vi "Add Output.vi"(0 "PainOutputTerminal in":refnum<class "PainOutputTerminal.lvclass">, 5 "Comiplation message":T1[](array[typedef]), 11 "error in (no error)":errorcluster) -> (4 "PainOutputTerminal out":refnum<class "PainOutputTerminal.lvclass">, 15 "error out":errorcluster)   [LabVIEW 2019, in "PainOutputTerminal.lvclass"]
uses:
  PainOutputTerminal.lvclass
  common/function utils/Validate_message.ctl
  common/function utils/Validate_MessageStatus.ctl
  PainOutputTerminal.lvclass/PainOutputTerminal.ctl
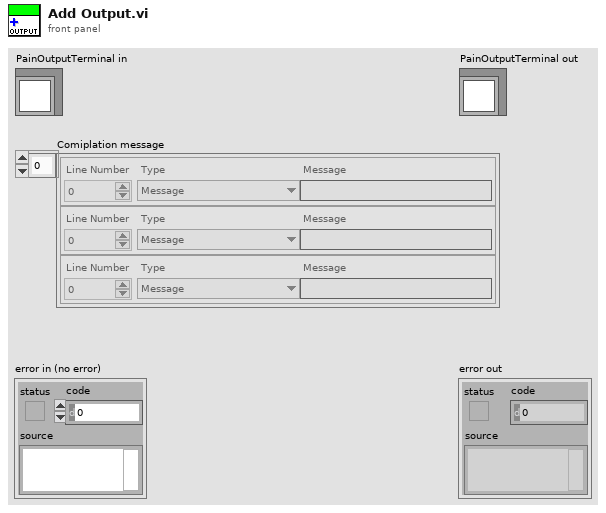
[diagram p1: front panel]
types:
  T1 = typedef "Validate_message.ctl" = cluster{"Line Number":i64, "Type":T2, "Message":string}
  T2 = typedef "Validate_MessageStatus.ctl" = enum16{"Message", "Warning", "Error"}
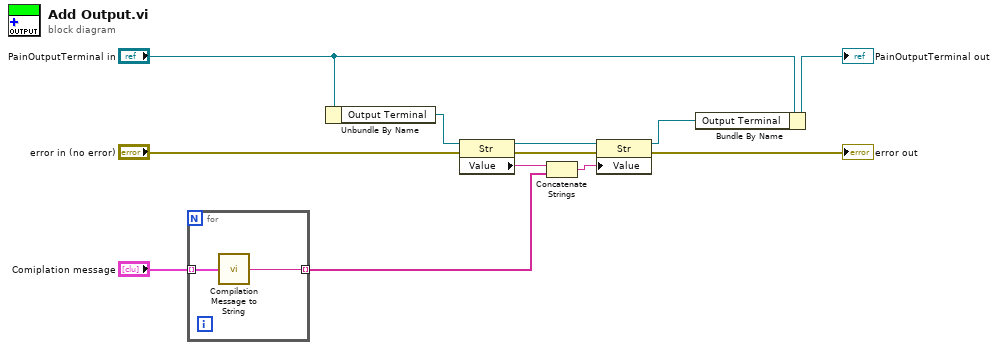
[diagram p0: block diagram]
diagram:
  n1 = for {
    tunnel: "Comiplation message" -> [w14] mode=indexing
    tunnel: [w13] -> w10 mode=indexing
    n2 = call "Compilation Message to String.vi"("Message"=w14) -> ("Messgae"=w13:string)  [unwired: 4 in]
  }
  n3 = Unbundle By Name("PainOutputTerminal in") -> ("Output Terminal"=w8:refnum<vi>)
  n4 = property class="Str"(reference=w8, error in="error in (no error)") -> (reference out=w6:refnum<vi>, error out=w9:errorcluster, "Value"=w2:string)
  n5 = Concatenate Strings(w2, w10) -> (w1:string)
  n6 = property class="Str"(reference=w6, error in=w9, "Value"=w1) -> (reference out=w5:refnum<vi>, error out=→"error out":errorcluster)
  n7 = Bundle By Name(cluster="PainOutputTerminal in", "Output Terminal"=w5) -> (→"PainOutputTerminal out":refnum<class "PainOutputTerminal.lvclass">)
